vi "To JSON Tree.vi"(8 "error in (no error)":errorcluster, 11 "params in":refnum<class "params.lvclass">) -> (0 "error out":errorcluster, 2 "JSON Tree Out":variant, 3 "params out":refnum<class "params.lvclass">)   [LabVIEW 2015, in "params.lvclass"]
uses:
  params.lvclass
  params.lvclass/params.ctl
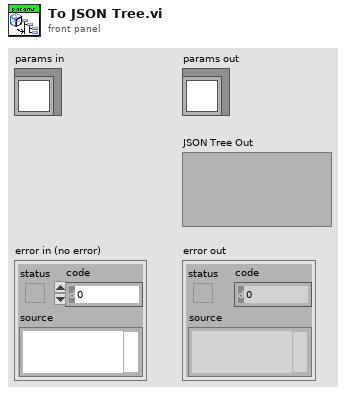
[diagram p1: front panel]
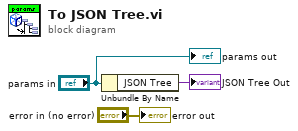
[diagram p0: block diagram]
diagram:
  n1 = Unbundle By Name("params in") -> ("JSON Tree"=→"JSON Tree Out":variant)
  "error out" <- "error in (no error)"
  "params out" <- "params in"
